vi "charge_controller.vi"(6 "Reset":bool, 7 "Parameters":T1={"Stimulus"={"Type"=enum."Off", "Delay"=0, "Amplitude"=[0.0, 0.0, 0.0], "Injection point"=enum."Total pose", "Closed loop"=FALSE, "Offset"=[0.0, 0.0, 0.0], "Tip -> world"=TRUE}, "Goal Filter A"={"Lower Fc"=0.0, "Lower Q"=0.15, "Scale factor"=0.0, "Upper Fc"=0.0075, "Upper Q"=0.01, "Manip zeroing"=0.001, "Speedup max"=150.0, "Speedup thresh"=5.0, "Speedup nonlin"=3.0, "V limit"=300.0, "V limit range"=300.0}, "Mode controls"={"Hold"=FALSE, "Cancellation"=FALSE, "Goal filter"=FALSE, "Trigger"=FALSE}, "Manipulator type"=enum."Current piezo", "Manipulator calibration"={"Inverse Kinematics"=[[-0.4736411481566654, -0.25724305819165183, -1.1087933259307599], [0.296735958809338, -0.258643951607561, -1.0971603505753995], [-0.043664688535758014, 0.44635679599468125, -1.1035515399424176]], "Handle transform"=[[3.281333089700394, 0.23462731743748497, 0.17832137948371765, -8265.081657965618], [-0.20249098046098263, 2.6933210343964133, -0.2815002765708058, -33565.66155248382], [-0.14581170473284072, 0.6821648518522063, 0.8833544952169589, 26862.18782130476], [-1.1202010727438122e-18, 5.861467994999758e-19, 1.760134464394436e-18, 0.999999999999992]], "Tip offset"=[0.0, 0.0, 36200.0], "Probe calibration"=[], "Pivot position"=[0.0, 0.0, -11360.0], "Axial filter"={"filter structure"=enum."IIR 2nd Order", "Reverse Coefficients"=[0.0, 0.0], "Forward Coefficients"=[1.0, 0.0, 0.0]}, "Lateral filter"={"filter structure"=enum."IIR 2nd Order", "Reverse Coefficients"=[0.0, 0.0], "Forward Coefficients"=[1.0, 0.0, 0.0]}}, "Charge piezo"={"Capacitance"=4e-08, "V min"=-235.0, "V max"=50.0, "- margin"=465.0, "+ margin"=0.001, "I max"=40000.0, "I sat"=90000000.0, "R series"=5.0, "R shunt"=1000.0, "Fault V"=0.0, "Start Fault V"=0.0, "Start Cycles"=0, "Prop gain"=1e-06, "Int gain"=0.0, "Diff gain"=0.0}, "Network"={"Remote Host"="192.168.1.3", "Send Status"=TRUE, "Send Port"=0, "Recv Commands"=FALSE, "Recv Port"=0}, "Goal Filter B"={"Lower Fc"=1.0, "Lower Q"=2.0, "Scale factor"=61557.0, "Upper Fc"=20.0, "Upper Q"=61557.0, "Manip zeroing"=2.0, "Speedup max"=1.0, "Speedup thresh"=300.0, "Speedup nonlin"=3.0, "V limit"=300.0, "V limit range"=300.0}, "Cancellation"={"Bandwidth"=0.0, "Delay"=0, "Stack travel"=0.0, "Saturation pos"=0.0075, "Slew Limit"=0.01, "Turnoff zeroing"=0.001, "Bypass"=FALSE}, "Transition time"=3.0} {"Transition time" format="%_3f"; "Cancellation"."Slew Limit" format="%#_3p"; "Cancellation"."Saturation pos" format="%#.1f"; "Cancellation"."Stack travel" format="%#.1f"; "Cancellation"."Turnoff zeroing" format="%#_6e"; "Cancellation"."Delay" step=1; "Cancellation"."Bandwidth" min=10 max=1000 step=10; "Goal Filter B"."V limit range" format="%_3p"; "Goal Filter B"."V limit" format="%_3p"; "Goal Filter B"."Speedup nonlin" format="%_3p"; "Goal Filter B"."Upper Q" format="%_3f"; "Goal Filter B"."Upper Fc" format="%_3p"; "Goal Filter B"."Lower Q" format="%_3f"; "Goal Filter B"."Speedup thresh" format="%_3p"; "Goal Filter B"."Speedup max" format="%_3p"; "Goal Filter B"."Manip zeroing" format="%_3p"; "Goal Filter B"."Scale factor" format="%_3f"; "Goal Filter B"."Lower Fc" format="%_3p"; "Charge piezo"."I sat" format="%#_6p"; "Charge piezo"."+ margin" format="%#_6p"; "Charge piezo"."- margin" format="%#_6p"; "Charge piezo"."Start Fault V" format="%#_6p"; "Charge piezo"."R shunt" format="%#_6p"; "Charge piezo"."Prop gain" format="%#_6p"; "Charge piezo"."Fault V" format="%#_6p"; "Charge piezo"."I max" format="%#_6p"; "Charge piezo"."Diff gain" format="%#_6p"; "Charge piezo"."Int gain" format="%#_6p"; "Charge piezo"."R series" format="%#_6p"; "Charge piezo"."Capacitance" format="%#_6p"; "Manipulator calibration"."Probe calibration" format="%#.1f"; "Manipulator calibration"."Handle transform" format="%#_3f"; "Manipulator calibration"."Inverse Kinematics" format="%#_3f"; "Goal Filter A"."V limit range" format="%_3p"; "Goal Filter A"."V limit" format="%_3p"; "Goal Filter A"."Speedup nonlin" format="%_3p"; "Goal Filter A"."Upper Q" format="%_3f"; "Goal Filter A"."Upper Fc" format="%_3p"; "Goal Filter A"."Lower Q" format="%_3f"; "Goal Filter A"."Speedup thresh" format="%_3p"; "Goal Filter A"."Speedup max" format="%_3p"; "Goal Filter A"."Manip zeroing" format="%_3p"; "Goal Filter A"."Scale factor" format="%_3f"; "Goal Filter A"."Lower Fc" format="%_3p"; "Stimulus"."Offset" step=100; "Stimulus"."Amplitude" step=100; "Stimulus"."Delay" step=100}, 9 "Stack voltage":sgl[](array[numeric]) format="%#.1f", 11 "Desired position":sgl[](array[numeric]) format="%#.1f") -> (0 "Saturation":bool[](array[boolean]), 1 "Slew limit":bool[](array[boolean]), 2 "Output current (ma)":sgl[](array[numeric]) format="%.2f", 3 "Stack positions":sgl[](array[numeric]) format="%#.1f")   [LabVIEW 2010]
uses:
  testing/Micron params.ctl
  testing/stimulus.ctl
  testing/injection_point.ctl
  filtering/goal_filter_parms.ctl
  testing/mode_conrols.ctl
  testing/manipulator_cal.ctl
  <vilib>/Analysis/Matrix/Datatypes/RealMatrix.ctl
  asap/labview/testing/probe_calibration.ctl
  Charge controller params.ctl
  host/network_params.ctl
  cancellation/im_control_params.ctl
  <vilib>/Analysis/Matrix/NI_Matrix.lvlib
panel:
  in  "Velocity Stack Gain":sgl
  in  "Velocity Current Gain":sgl
  out "Startup over":bool
  in  "Charge integrator":sgl[](array[numeric])=[0.0, 0.0, 0.0] format="%#_3p"
  in  "Last charge":sgl[](array[numeric])=[0.0, 0.0, 0.0] format="%#_3p"
  # "Locals:"
  # "New charge we expect after this cycle (C)."
  # "Our estimate of the net charge in the piezos before the previous cycle (C).  This lags \"Charge integrator\" by one cycle.  We need this to compute V error, since the output for prev cycle is synchronized with input for this cycle."
  # "True if startup mode (calibration of offset current) is finished."
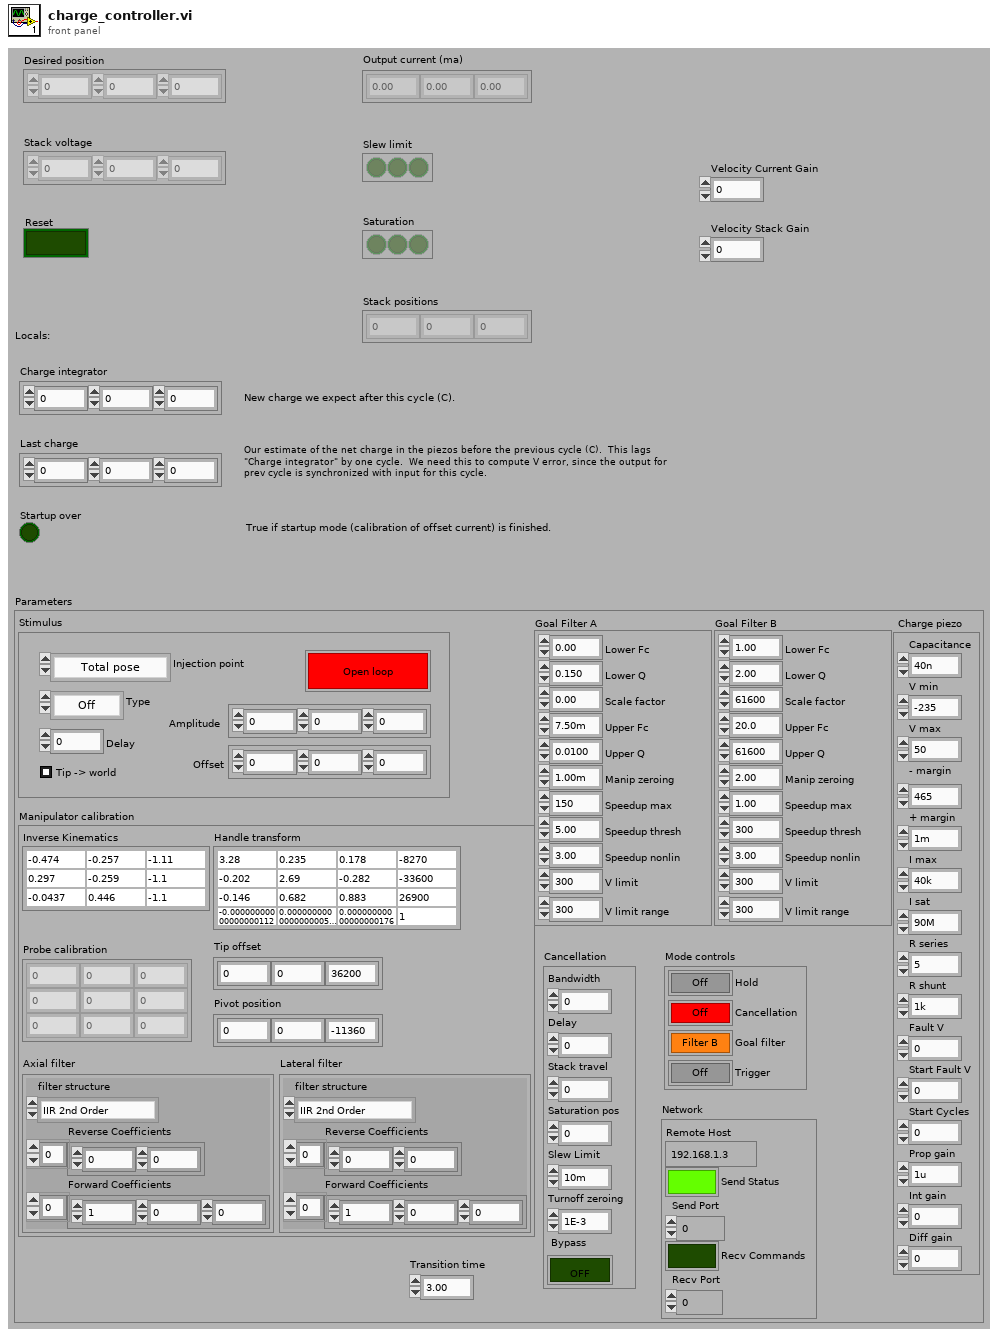
[diagram p1: front panel]
types:
  T1 = typedef "Micron params.ctl" = cluster{"Stimulus":T2, "Goal Filter A":T4, "Mode controls":T5, "Manipulator type":enum16{"Current piezo", "Voltage piezo"}, "Manipulator calibration":T6, "Charge piezo":T9, "Network":T10, "Goal Filter B":T4, "Cancellation":T11, "Transition time":sgl}
  T2 = typedef "stimulus.ctl" = cluster{"Type":enum16{"Off", "Step", "Sine", "Triangle", "Arbitrary"}, "Delay":i32, "Amplitude":sgl[], "Injection point":T3, "Closed loop":bool, "Offset":sgl[], "Tip -> world":bool}
  T3 = typedef "injection_point.ctl" = enum16{"Total pose", "V limiter", "Goal position", "Tip error (manip)", "Inverse kin", "Controller", "Stack position", "Stack drive", "DAC"}
  T4 = typedef "goal_filter_parms.ctl" = cluster{"Lower Fc":sgl, "Lower Q":sgl, "Scale factor":sgl, "Upper Fc":sgl, "Upper Q":sgl, "Manip zeroing":sgl, "Speedup max":sgl, "Speedup thresh":sgl, "Speedup nonlin":sgl, "V limit":sgl, "V limit range":sgl}
  T5 = typedef "mode_conrols.ctl" = cluster{"Hold":bool, "Cancellation":bool, "Goal filter":bool, "Trigger":bool}
  T6 = typedef "manipulator_cal.ctl" = cluster{"Inverse Kinematics":T7, "Handle transform":T7, "Tip offset":sgl[], "Probe calibration":T8, "Pivot position":sgl[], "Axial filter":cluster{"filter structure":enum32{"IIR 2nd Order", "IIR 4th Order"}, "Reverse Coefficients":dbl[], "Forward Coefficients":dbl[]}, "Lateral filter":cluster{"filter structure":enum32{"IIR 2nd Order", "IIR 4th Order"}, "Reverse Coefficients":dbl[], "Forward Coefficients":dbl[]}}
  T7 = typedef "NI_Matrix.lvlib/RealMatrix.ctl" = dbl[][]
  T8 = typedef "probe_calibration.ctl" = sgl[][]
  T9 = typedef "Charge controller params.ctl" = cluster{"Capacitance":sgl, "V min":sgl, "V max":sgl, "- margin":sgl, "+ margin":sgl, "I max":sgl, "I sat":sgl, "R series":sgl, "R shunt":sgl, "Fault V":sgl, "Start Fault V":sgl, "Start Cycles":i32, "Prop gain":sgl, "Int gain":sgl, "Diff gain":sgl}
  T10 = typedef "network_params.ctl" = cluster{"Remote Host":string, "Send Status":bool, "Send Port":u16, "Recv Commands":bool, "Recv Port":u16}
  T11 = typedef "im_control_params.ctl" = cluster{"Bandwidth":sgl, "Delay":i32, "Stack travel":sgl, "Saturation pos":sgl, "Slew Limit":sgl, "Turnoff zeroing":sgl, "Bypass":bool}
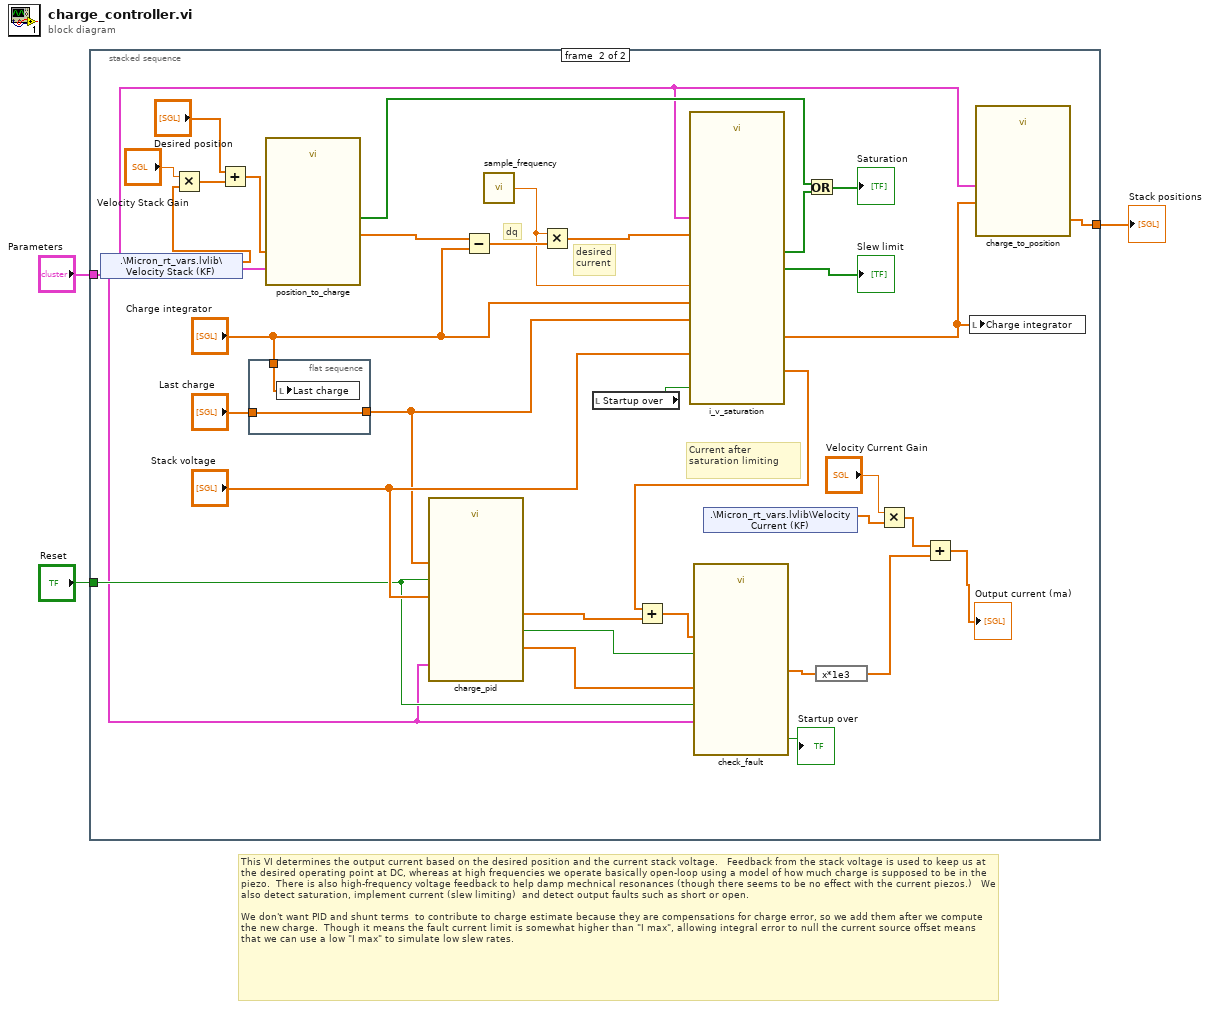
[diagram p0: block diagram]
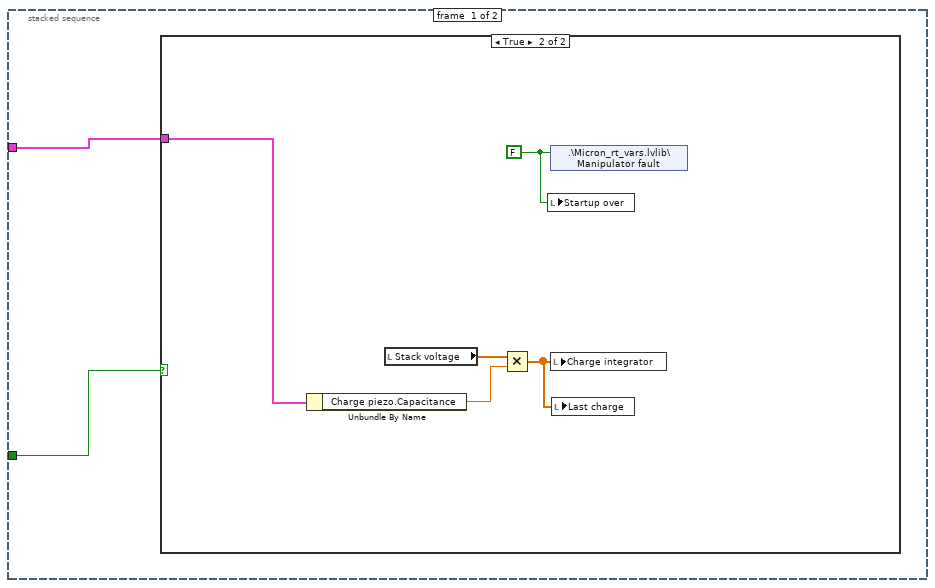
[diagram p2: hidden frame]
diagram:
  # "This VI determines the output current based on the desired position and the current stack voltage.   Feedback from the stack voltage is used to keep us at the desired operating point at DC, whereas at high frequencies we operate basically open-loop using a model of how much charge is supposed to be in the piezo.  There is also high-frequency voltage feedback to help damp mechnical resonances (though there seems to be no effect with the current piezos.)   We also detect saturation, implement current (slew limiting)  and detect output faults such as short or open.\n\nWe don't want PID and shunt terms  to contribute to charge estimate because they are compensations for charge error, so we add them after we compute the new charge.  Though it means the fault current limit is somewhat higher than \"I max\", allowing integral error to null the current source offset means that we can use a low \"I max\" to simulate low slew rates."
  n1 = stacked-sequence {
    tunnel: "Reset" -> [w5 w38]
    tunnel: "Parameters" -> [w4 w29]
    tunnel: [_ w21] -> w1
    frame #0 {
      n2 = case shown="True" w5 {
        tunnel: w4 -> [_ w8]
        frame False {
        }
        frame True {
          w6 = FALSE ("Manipulator fault")
          n3 = Unbundle By Name(w8) -> ("Charge piezo.Capacitance"=w9:sgl)
          n4 = local read "Stack voltage"() -> (w10:sgl[])
          n5 = Multiply(x=w10, y=w9) -> (x*y=w7:sgl[])
          n6 = local write "Startup over"(w6) -> ()
          n7 = shared-variable ".\\Micron_rt_vars.lvlib\\Manipulator fault"(w6) -> ()  [unwired: 2 out]
          n8 = local write "Charge integrator"(w7) -> ()
          n9 = local write "Last charge"(w7) -> ()
        }
      }
    }
    frame #1 {
      # "Current after saturation limiting"
      # "desired\ncurrent"
      # "dq"
      n10 = shared-variable ".\\Micron_rt_vars.lvlib\\Velocity Stack (KF)"() -> (w15:sgl[])  [unwired: 2 out]
      n11 = Multiply(x="Velocity Stack Gain", y=w15) -> (x*y=w11:sgl[])
      n12 = Add(x="Desired position", y=w11) -> (x+y=w13:sgl[])
      n13 = flat-sequence {
        tunnel: "Charge integrator" -> [w46]
        tunnel: [w45] -> w22
        tunnel: "Last charge" -> [w45]
        frame #0 {
          n14 = local write "Last charge"(w46) -> ()
        }
      }
      n15 = call "position_to_charge.vi"("Parameters"=w29, "Desired position"=w13) -> ("Saturation"=w39:bool[], "Charge goal"=w43:sgl[])  [unwired: 8 out]
      n16 = call "charge_pid.vi"("Parameters"=w29, "Reset"=w38, "Stack voltage"="Stack voltage", "Charge estimate"=w22) -> ("Voltage error"=w37:sgl[], "Result"=w26:sgl[], "Integrator saturation"=w36:bool)  [unwired: 2 in, 3 out]
      n17 = Subtract(x=w43, y="Charge integrator") -> (x-y=w44:sgl[])
      n18 = call "sample_frequency.vi"() -> ("Sample frequency"=w32:sgl)
      n19 = Multiply(x=w32, y=w44) -> (x*y=w35:sgl[])
      n20 = local read "Startup over"() -> (w24:bool)
      n21 = call "i_v_saturation.vi"("Parameters"=w29, "Stack voltage"="Stack voltage", "I in"=w35, "Sample frequency"=w32, "Current charge"="Charge integrator", "Startup over"=w24, "Last charge"=w22) -> ("Saturation"=w40:bool[], "Slew limit"=→"Slew limit":bool[], "New charge"=w28:sgl[], "I out"=w27:sgl[])  [unwired: 1 out]
      n22 = Add(x=w27, y=w26) -> (x+y=w33:sgl[])
      n23 = call "check_fault.vi"("Reset"=w38, "Parameters"=w29, "V error"=w37, "Integrator saturation"=w36, "I in"=w33) -> ("Startup over"=→"Startup over":bool, "I out"=w34:sgl[])  [unwired: 5 out]
      n24 = shared-variable ".\\Micron_rt_vars.lvlib\\Velocity Current (KF)"() -> (w19:sgl[])  [unwired: 2 out]
      n25 = Or(x=w39, y=w40) -> (x .or. y?=→"Saturation":bool[])
      n26 = expression code="x*1e3"(w34) -> (w17:sgl[])
      n27 = Multiply(x="Velocity Current Gain", y=w19) -> (x*y=w18:sgl[])
      n28 = Add(x=w18, y=w17) -> (x+y=→"Output current (ma)":sgl[])
      n29 = local write "Charge integrator"(w28) -> ()
      n30 = call "charge_to_position.vi"("Parameters"=w29, "Charge estimate"=w28) -> ("Stack positions"=w21:sgl[])  [unwired: 9 out]
    }
  }
  "Stack positions" <- w1
